vi "XYZ Get Status.vi"(0 "LSID in":i32, 11 "error in (no error)":errorcluster) -> (4 "Controller Status":string, 6 "Axis Status":T1(array[ring]), 8 "Motion Done?":bool, 10 "Axis Status":string, 15 "error out":errorcluster)   [LabVIEW 2014]
uses:
  <userlib>/Tango_DLL/Tango_DLL.lvlib
panel:
  # "LICENSED MATERIALS – PROPERTY OF IBM\nCopyright IBM Corp. 2016,\nALL RIGHTS RESERVED"
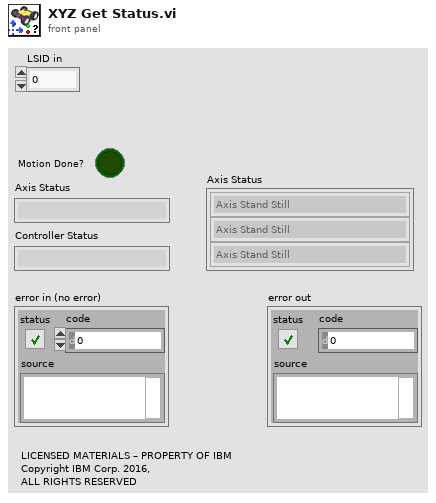
[diagram p1: front panel]
types:
  T1 = enum16{"Axis Stand Still", "Axis in Motion", "Axis Disabled", "Joystick on", "Axis in Closed Loop", "Return Message After Calibration", "Calibration Error", "Return Message after Travel", "Setup Mode", "Timeout", "Status Unknown"}[]
  T2 = enum16{"Axis Stand Still", "Axis in Motion", "Axis Disabled", "Joystick on", "Axis in Closed Loop", "Return Message After Calibration", "Calibration Error", "Return Message after Travel", "Setup Mode", "Timeout", "Status Unknown"}
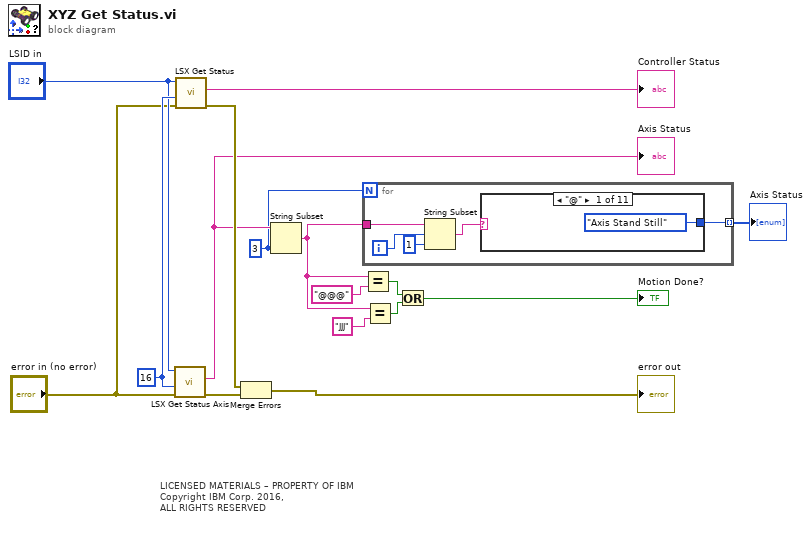
[diagram p0: block diagram]
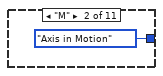
[diagram p2: hidden frame]
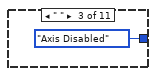
[diagram p3: hidden frame]
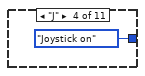
[diagram p4: hidden frame]
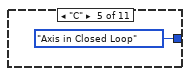
[diagram p5: hidden frame]
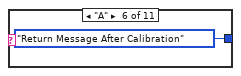
[diagram p6: hidden frame]
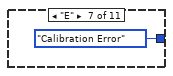
[diagram p7: hidden frame]
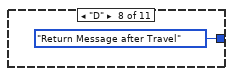
[diagram p8: hidden frame]
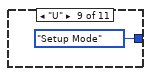
[diagram p9: hidden frame]
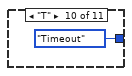
[diagram p10: hidden frame]
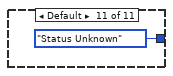
[diagram p11: hidden frame]
diagram:
  w2 = 3 ("length (rest)")
  w16 = 16 ("lMaxLen")
  # "LICENSED MATERIALS – PROPERTY OF IBM\nCopyright IBM Corp. 2016,\nALL RIGHTS RESERVED"
  n1 = call <userlib>:"LSX Get Status Axis.vi"("error in (no error)"="error in (no error)", "lMaxLen"=w16, "lLSID"="LSID in") -> ("error out"=w15:errorcluster, "pcStatusAxisStr out"=w5:string)  [unwired: 6 in, 1 out]
  "Axis Status" <- w5
  n2 = call <userlib>:"LSX Get Status.vi"("error in (no error)"="error in (no error)", "lMaxLen"=w16, "lLSID"="LSID in") -> ("error out"=w6:errorcluster, "pcStat out"=→"Controller Status":string)  [unwired: 6 in, 1 out]
  n3 = Merge Errors(w6, w15) -> (→"error out":errorcluster)
  n4 = String Subset(string=w5, length (rest)=w2) -> (substring=w3:string)  [unwired: 1 out]
  n5 = for {
    N: w2 -> [_]
    tunnel: [w21] -> w1 mode=indexing
    tunnel: w3 -> [w20]
    i -> [w19]
    n6 = String Subset(string=w20, offset (0)=w19, length (rest)=1 ("length (rest)")) -> (substring=w17:string)
    n7 = case shown="\"@\"" w17 {
      tunnel: [T2."Axis Stand Still" ("Status 2") T2."Axis in Motion" ("Status 2") T2."Axis Disabled" ("Status 2") T2."Joystick on" ("Status 2") T2."Axis in Closed Loop" ("Status 2") T2."Return Message After Calibration" ("Status 2") T2."Calibration Error" ("Status 2") T2."Return Message after Travel" ("Status 2") T2."Setup Mode" ("Status 2") T2."Timeout" ("Status 2") T2."Status Unknown" ("Status 2")] -> w21
      frame "@" {
      }
      frame "M" {
      }
      frame " " {
      }
      frame "J" {
      }
      frame "C" {
      }
      frame "A" {
      }
      frame "E" {
      }
      frame "D" {
      }
      frame "U" {
      }
      frame "T" {
      }
      frame Default {
      }
    }
  }
  "Axis Status" <- w1
  n8 = Equal?(x=w3, y="@@@") -> (x = y?=w14:bool)
  n9 = Equal?(x=w3, y="JJJ") -> (x = y?=w13:bool)
  n10 = Or(x=w14, y=w13) -> (x .or. y?=→"Motion Done?":bool)
